vi "BLM_ManualControl.vi"() -> ()   [LabVIEW 2020]
doc: "To start rotations:\n\nSelect The Motor (BLM) address\nRun this VI\nClick Test connection button\nClick INITIALIZE button \n (It is assumed that a BLM controller should be initialized only once: immediately after it is turned on. \n E.g., usually there is no need to initialize if you rebooted computer, but kept the motor controller on,\n the motor was connected to the controller and you wish to continue using current position counting. \n Initialization occurs only if the current motor position is equal to zero.) \nClick READ BLM position button\nSelect desired MODE, SPEED, and Distance (or Final Position, depends on the MODE) value\nClick RUN BLM button\n\nSET POSITION button does not affect actual sample/motor position, but changes the position value\nin the controller memory. Thus, it allows to assign any value to the current motor position.\n\nSee also:\nhttps://opswiki.magnet.fsu.edu/wiki/pages/K7Q8u4C4s9/Rotating_probes_equipped_with_Brushless_Motors_BLMs.html\n\nNHMFL; A.Suslov; Feb 2012; updated Aug 2016"
panel:
  out "Error Out":errorcluster {"code" format="%.0x"}
  in  "MODE:":enum32{"ABSOLUTE", "INCREMENTAL"}(radio)=enum."INCREMENTAL"
  in  "Read Position":bool
  out "Test Results":string
  in  "Test Connection":bool
  out "BLM Position":dbl caption="BLM position\nincrement 0.045 \n (deg of BLM)" format="%.3f"
  in  "Parameter changed":bool
  in  "stop":bool
  in  "Set Position":bool
  in  "INITIALIZE":bool
  in  "Run":bool
  in  "New position":dbl caption="Distance:\nincrement 0.045 \n (deg of BLM)" step=0.045 format="%#.3g"
  in  "SPEED (rot/sec)\nincrement .0042":dbl=0.0294 min=0.0042 max=0.42 step=0.0042
  in  "MOTOR (BLM) Address":refnum<visa-resource-name>
  # "Select The Motor (BLM) address\nRun this VI\nClick Test connection button\nClick  INITIALIZE button \nClick  READ BLM position button\nSelect desired MODE, SPEED, and\n         Distance (or Final Position)\nClick RUN BLM button\n\nMore Help at File-> VI Propeties->\nDocumentation\nand Operations Wiki"
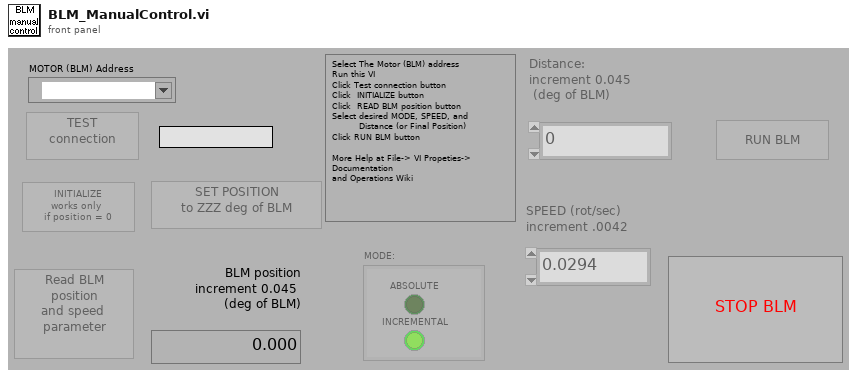
[diagram p1: front panel]
types:
  T1 = enum8{"Enabled", "Disabled", "Disabled and Grayed Out"}
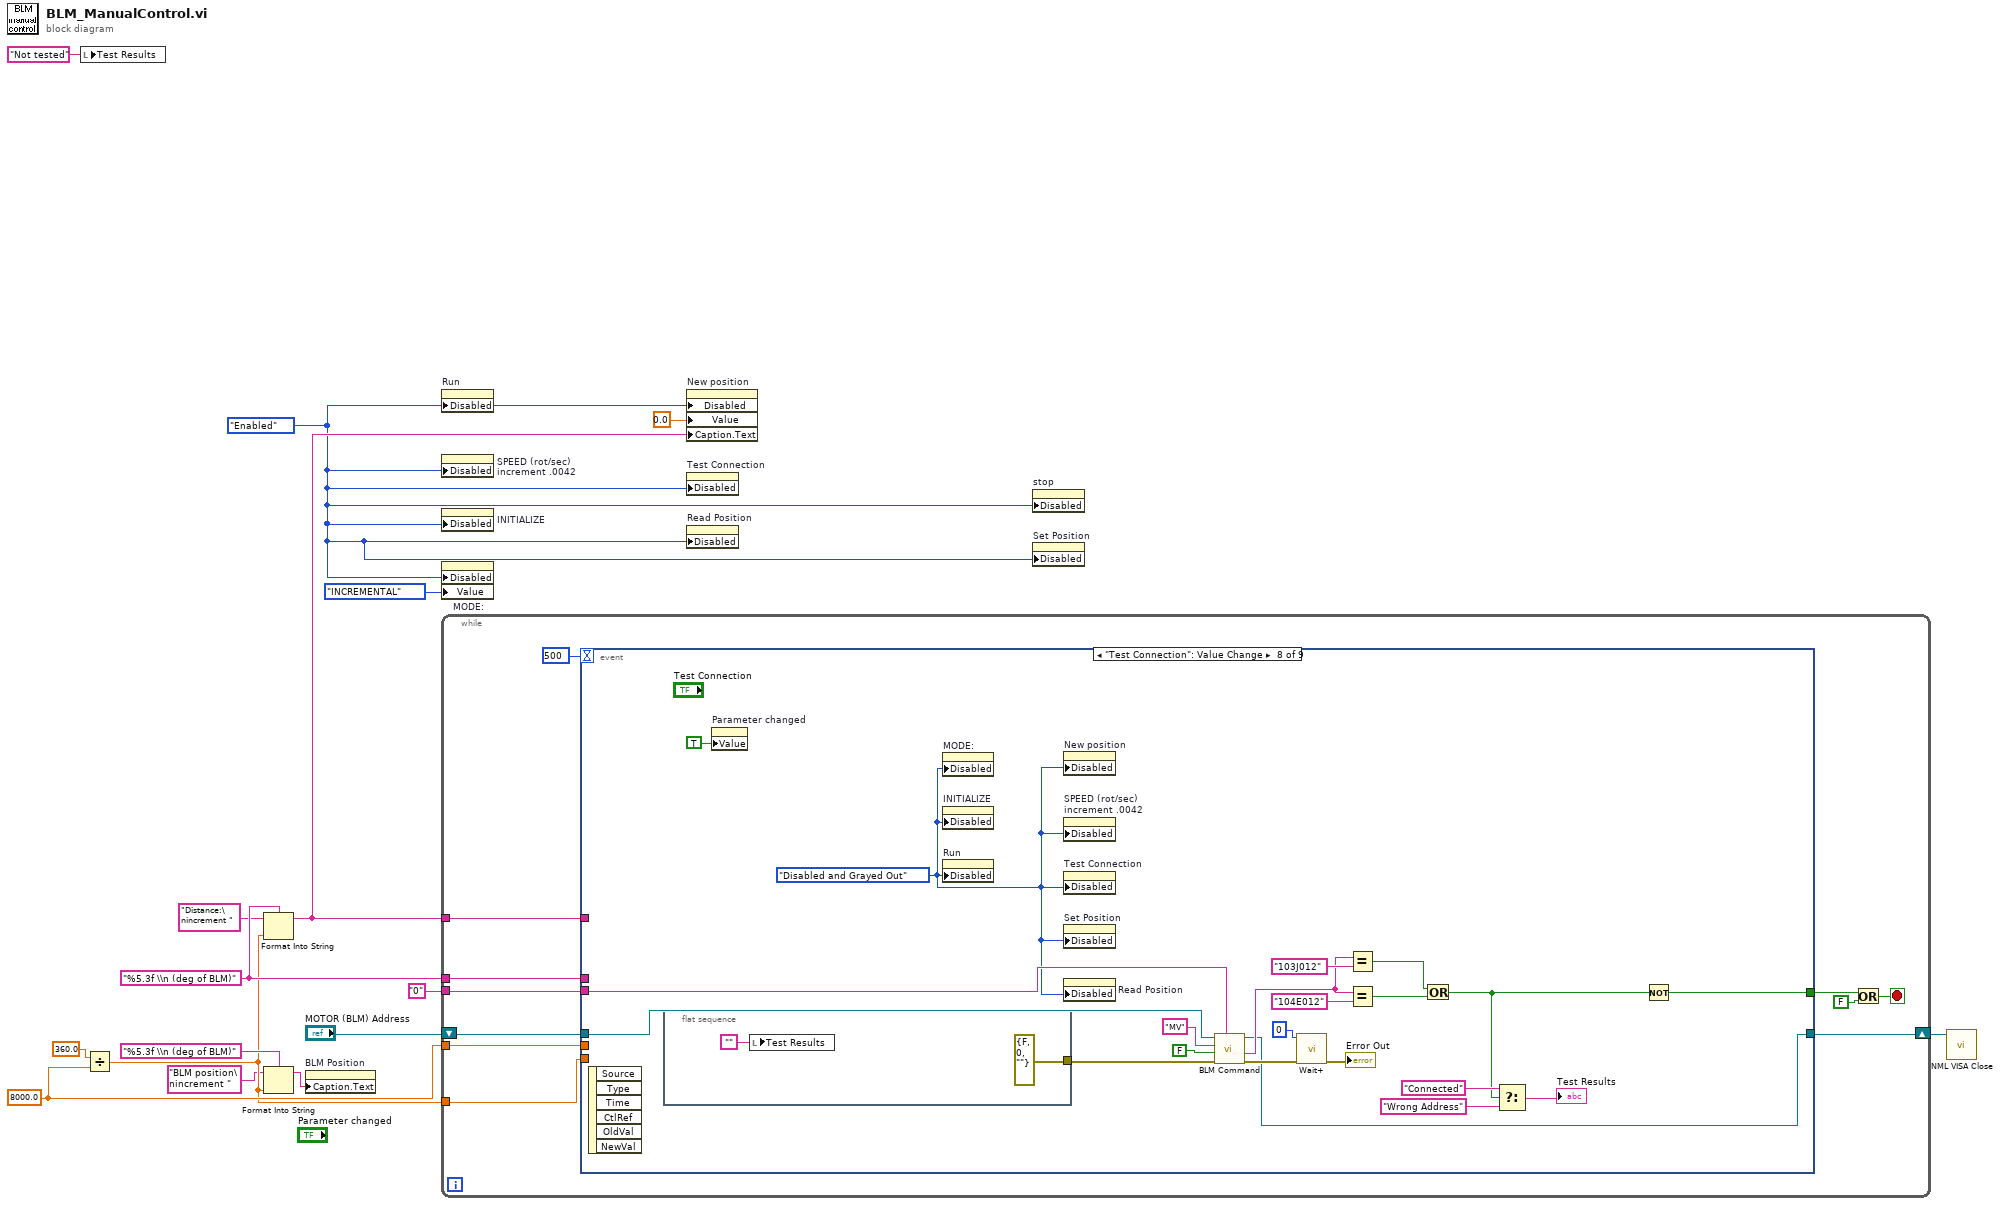
[diagram p0: block diagram]
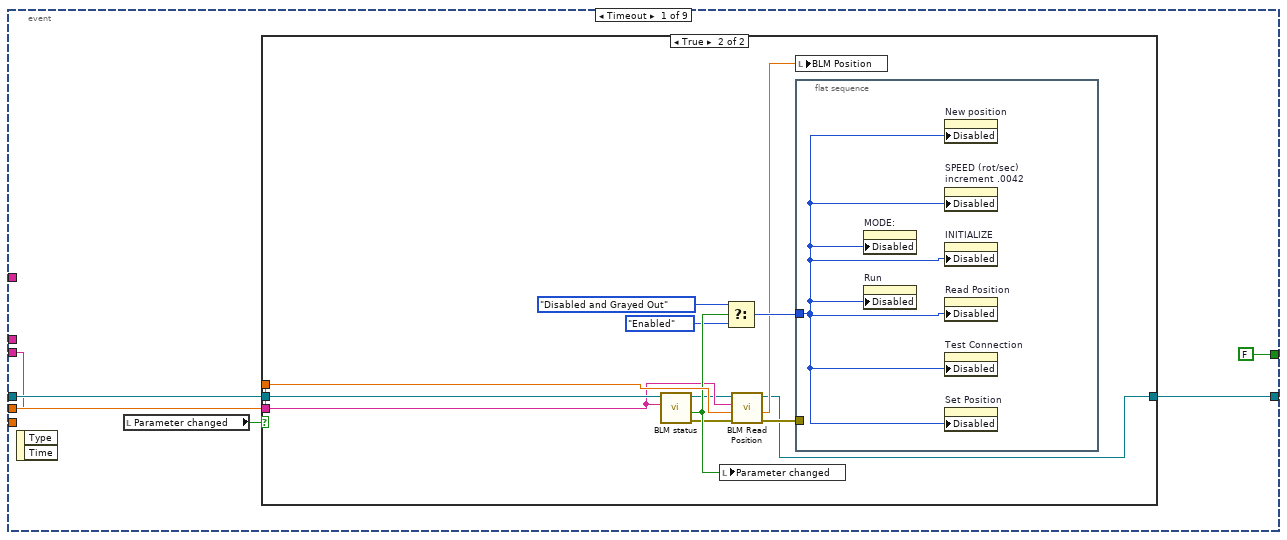
[diagram p2: hidden frame]
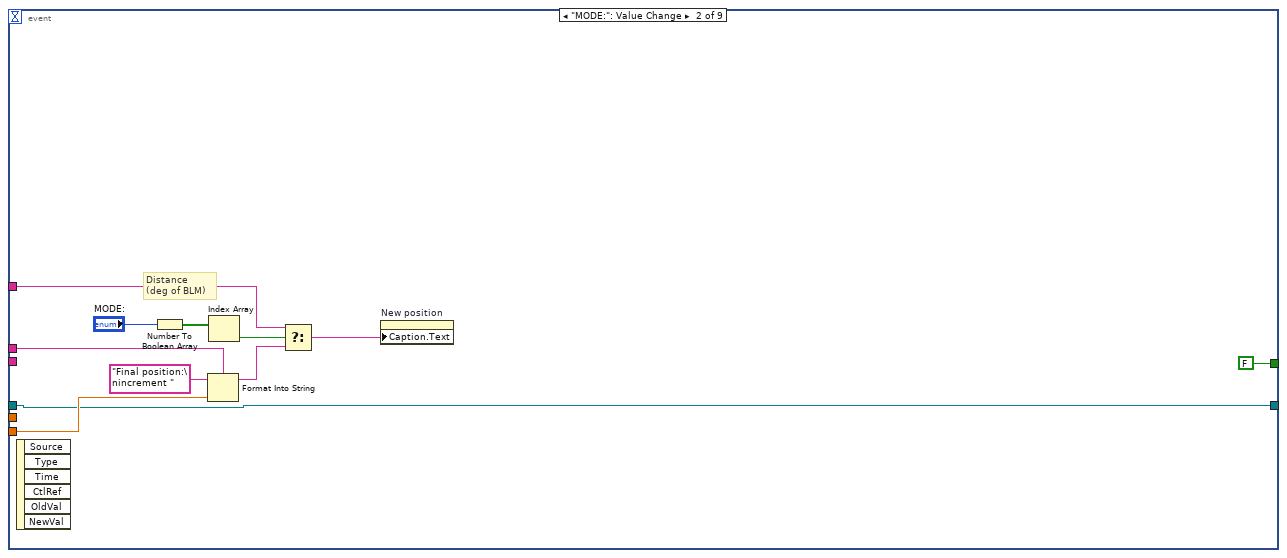
[diagram p4: hidden frame]
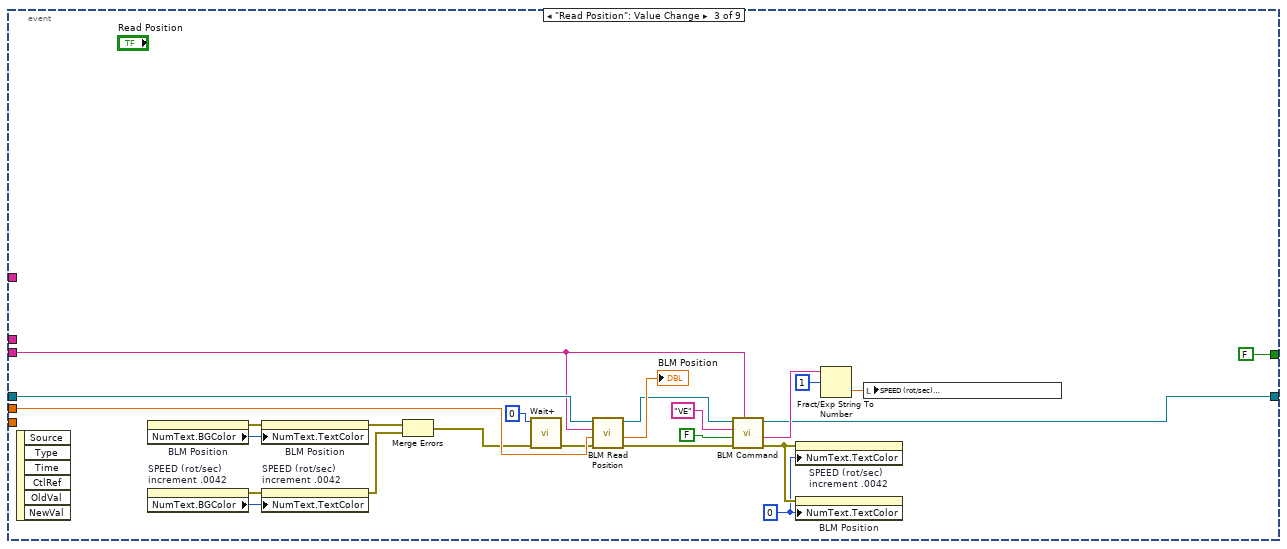
[diagram p5: hidden frame]
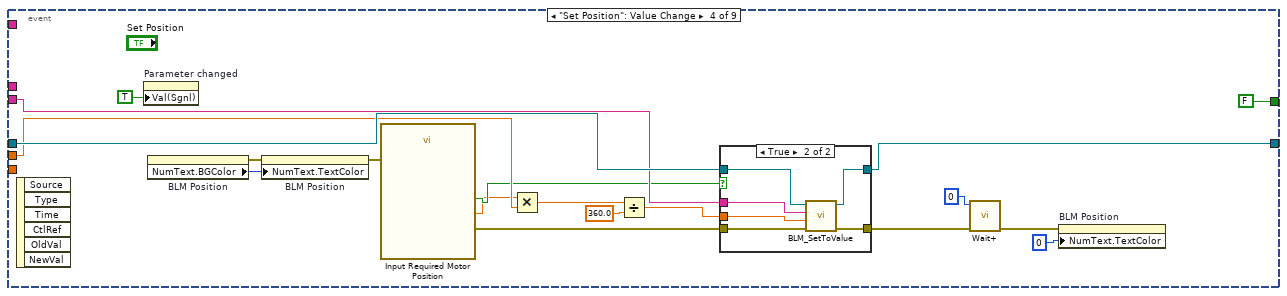
[diagram p6: hidden frame]
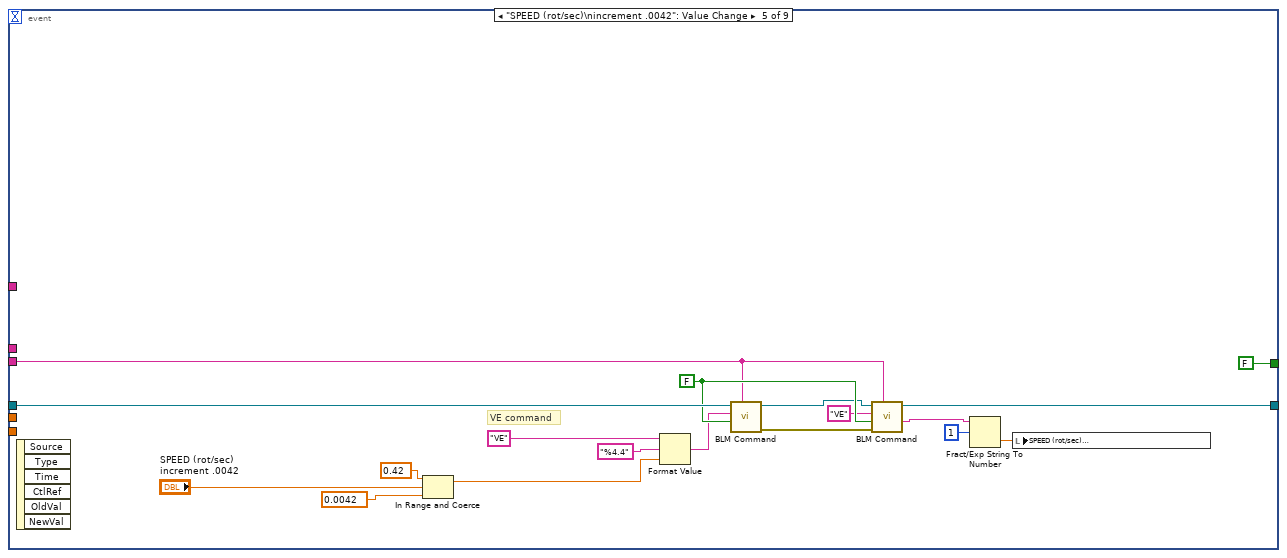
[diagram p8: hidden frame]
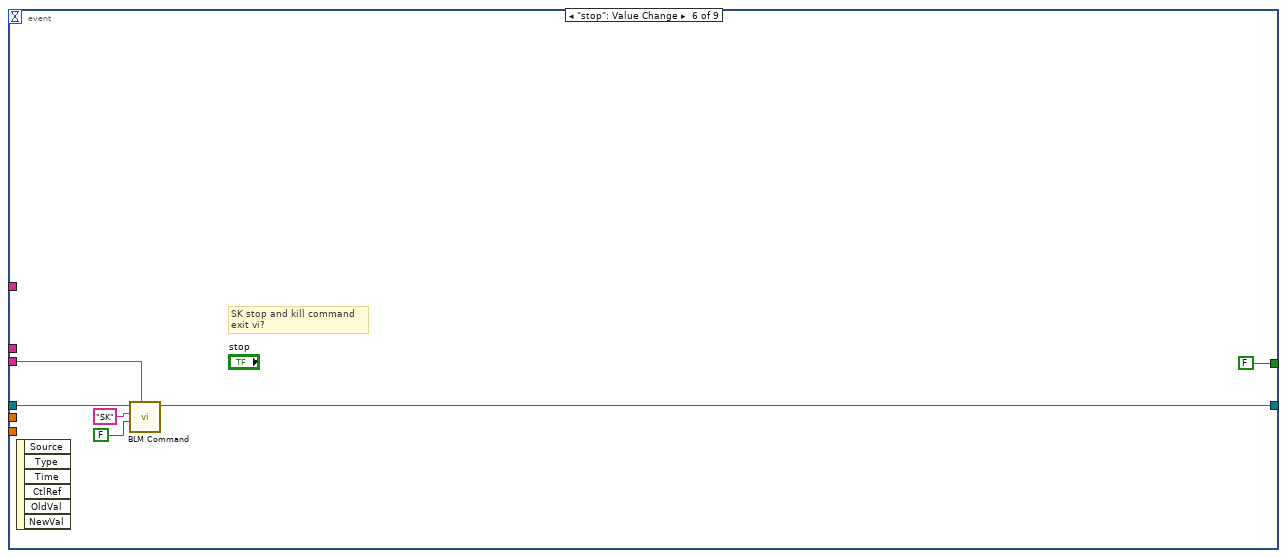
[diagram p9: hidden frame]
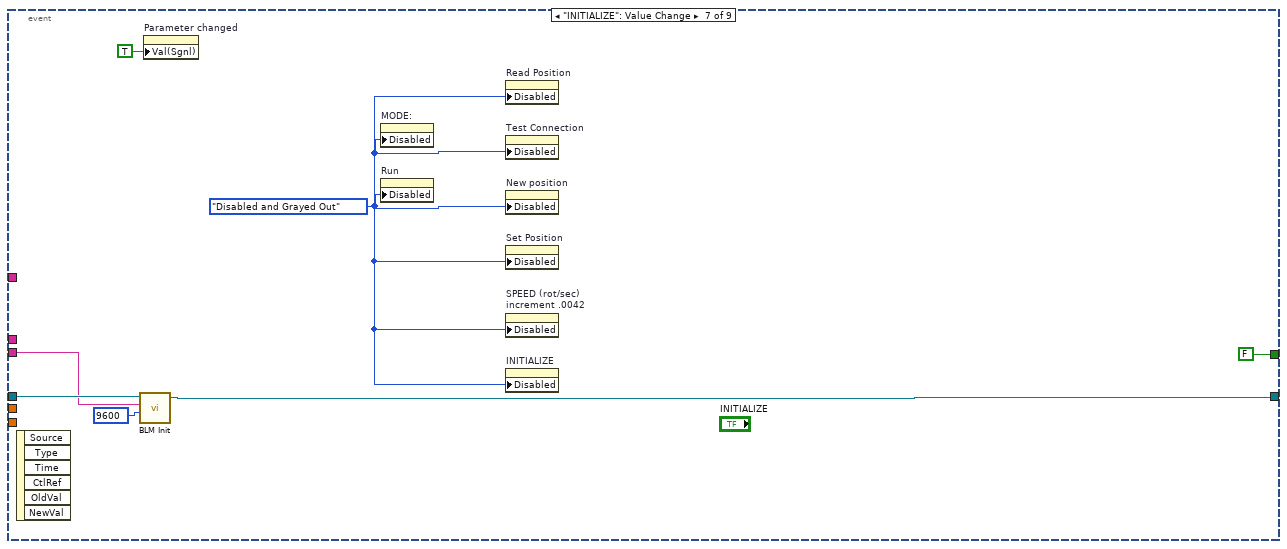
[diagram p10: hidden frame]
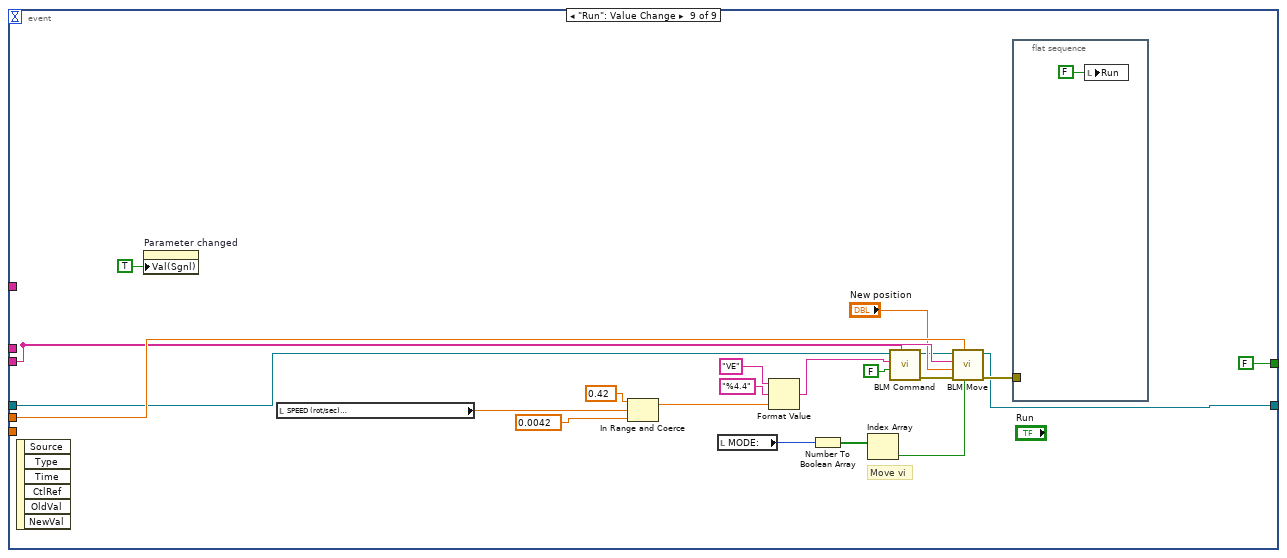
[diagram p11: hidden frame]
diagram:
  w3 = T1."Enabled" ("Disabled")
  w9 = "%5.3f \\n (deg of BLM)" ("format string")
  w11 = 8000.0 ("Steps/rot")
  n1 = local write "Test Results"("Not tested" ("s? t:f")) -> ()
  n2 = Divide(x=360.0, y=w11) -> (x/y=w6:dbl)
  n3 = Format Into String(format string=w9, initial string="Distance:\nincrement " ("Label.Text"), w6) -> (resulting string=w10:string)  [unwired: 1 in, 1 out]
  n4 = Format Into String(format string="%5.3f \\n (deg of BLM)", initial string="BLM position\nincrement ", w6) -> (resulting string=w7:string)  [unwired: 1 in, 1 out]
  n5 = property on="BLM Position" class="DigNum (strict)"("Caption.Text"=w7) -> ()  [unwired: 2 in, 2 out]
  n6 = property on="Run" class="Bool (strict)"("Disabled"=w3) -> ()  [unwired: 2 in, 2 out]
  n7 = property on="SPEED (rot/sec)\nincrement .0042" class="DigNum (strict)"("Disabled"=w3) -> ()  [unwired: 2 in, 2 out]
  n8 = property on="INITIALIZE" class="Bool"("Disabled"=w3) -> ()  [unwired: 2 in, 2 out]
  n9 = property on="MODE:" class="RadioBtnsControl (strict)"("Disabled"=w3, "Value"=enum32{"ABSOLUTE", "INCREMENTAL"}."INCREMENTAL" ("MODE:")) -> ()  [unwired: 2 in, 2 out]
  n10 = while {
    tunnel: w11 -> [w27]
    tunnel: w10 -> [w21]
    tunnel: "0" ("Motor Address") -> [w20]
    tunnel: w6 -> [w19]
    tunnel: w9 -> [w18]
    shift-right: [w17] -> w1
    shift-left: "MOTOR (BLM) Address" -> [w26]
    stop <- w23 stop-if-true
    n11 = event shown="[7] \"Test Connection\": Value Change" {
      selector: _ -> [_ _ _ _ _ _ _ _ _]
      dyn-events: _ -> [_ _ _ _ _ _ _ _ _]
      timeout: 500 -> [_ _ _ _ _ _ _ _ _]
      tunnel: w27 -> [w32 _ w82 w98 _ _ _ _ w184]
      tunnel: w26 -> [w33 w48 w81 w101 w127 w133 w139 w161 w183]
      tunnel: [FALSE FALSE FALSE FALSE FALSE FALSE FALSE w159 FALSE] -> w22
      tunnel: w21 -> [_ w57 _ _ _ _ _ _ _]
      tunnel: w20 -> [w30 _ w80 w99 w123 w130 w137 w157 w181]
      tunnel: w19 -> [_ w51 _ _ _ _ _ _ _]
      tunnel: w18 -> [_ w50 _ _ _ _ _ _ _]
      tunnel: [w28 w48 w59 w83 w110 w128 w134 w141 w164] -> w17
      event Timeout {
        n12 = event-data() -> ()  [unwired: 1 in, 2 out]
        n13 = local read "Parameter changed"() -> (w31:bool)
        n14 = case shown="True" w31 {
          tunnel: w33 -> [w34 w46]
          tunnel: w32 -> [_ w45]
          tunnel: w30 -> [_ w41]
          tunnel: [w34 w36] -> w28
          frame False {
          }
          frame True {
            n15 = call "BLM status.vi"("Motor Address"=w41, "Port Address"=w46) -> ("error out"=w40:errorcluster, "Motor is moving"=w44:bool, "Port Address Out"=w35:refnum<visa-resource-name>)  [unwired: 3 in]
            n16 = local write "Parameter changed"(w44) -> ()
            n17 = Select(t=T1."Disabled and Grayed Out" ("Disabled"), s=w44, f=T1."Enabled" ("Disabled")) -> (s? t:f=w43:T1)
            n18 = call "BLM Read Position.vi"("error in (no error)"=w40, "Steps/rot"=w45, "Motor Address"=w41, "Port Address"=w35) -> ("error out"=w39:errorcluster, "Response"=w42:dbl, "Port Address Out"=w36:refnum<visa-resource-name>)  [unwired: 1 out]
            n19 = local write "BLM Position"(w42) -> ()
            n20 = flat-sequence {
              tunnel: w43 -> [w47]
              tunnel: w39 -> [_]
              frame #0 {
                n21 = property on="MODE:" class="RadioBtnsControl (strict)"("Disabled"=w47) -> ()  [unwired: 2 in, 2 out]
                n22 = property on="Run" class="Bool (strict)"("Disabled"=w47) -> ()  [unwired: 2 in, 2 out]
                n23 = property on="New position" class="DigNum (strict)"("Disabled"=w47) -> ()  [unwired: 2 in, 2 out]
                n24 = property on="SPEED (rot/sec)\nincrement .0042" class="DigNum (strict)"("Disabled"=w47) -> ()  [unwired: 2 in, 2 out]
                n25 = property on="INITIALIZE" class="Bool"("Disabled"=w47) -> ()  [unwired: 2 in, 2 out]
                n26 = property on="Read Position" class="Bool"("Disabled"=w47) -> ()  [unwired: 2 in, 2 out]
                n27 = property on="Test Connection" class="Bool"("Disabled"=w47) -> ()  [unwired: 2 in, 2 out]
                n28 = property on="Set Position" class="Bool"("Disabled"=w47) -> ()  [unwired: 2 in, 2 out]
              }
            }
          }
        }
      }
      event "MODE:": Value Change {
        # "Distance  \n(deg of BLM)"
        n29 = event-data() -> ()  [unwired: 1 in, 6 out]
        n30 = Number To Boolean Array(number="MODE:") -> (Boolean array=w55:bool[])
        n31 = Format Into String(format string=w50, initial string="Final position:\nincrement " ("f"), w51) -> (resulting string=w53:string)  [unwired: 1 in, 1 out]
        n32 = Index Array(array=w55) -> (element=w54:bool)  [unwired: 1 in]
        n33 = Select(t=w57, s=w54, f=w53) -> (s? t:f=w58:string)
        n34 = property on="New position" class="DigNum (strict)"("Caption.Text"=w58) -> ()  [unwired: 2 in, 2 out]
      }
      event "Read Position": Value Change {
        w67 = u32 0 ("Numeric Text.Text Colors:Text Color")
        n35 = event-data() -> ()  [unwired: 1 in, 6 out]
        n36 = property on="BLM Position" class="DigNum (strict)"() -> (error out=w61:errorcluster, "NumText.BGColor"=w66:u32)  [unwired: 2 in, 1 out]
        n37 = property on="SPEED (rot/sec)\nincrement .0042" class="DigNum (strict)"() -> (error out=w62:errorcluster, "NumText.BGColor"=w65:u32)  [unwired: 2 in, 1 out]
        n38 = property on="BLM Position" class="DigNum (strict)"(error in=w61, "NumText.TextColor"=w66) -> (error out=w64:errorcluster)  [unwired: 1 in, 1 out]
        n39 = property on="SPEED (rot/sec)\nincrement .0042" class="DigNum (strict)"(error in=w62, "NumText.TextColor"=w65) -> (error out=w63:errorcluster)  [unwired: 1 in, 1 out]
        n40 = Merge Errors(w64, w63) -> (w68:errorcluster)
        n41 = call "Wait+.vi"("Error In"=w68, "milliseconds to wait"=u32 0 ("millisecond timer value")) -> ("Error Out"=w70:errorcluster)  [unwired: 4 in, 1 out]
        n42 = call "BLM Read Position.vi"("error in (no error)"=w70, "Steps/rot"=w82, "Motor Address"=w80, "Port Address"=w81) -> ("error out"=w72:errorcluster, "Response"=→"BLM Position":dbl, "Port Address Out"=w60:refnum<visa-resource-name>)  [unwired: 1 out]
        n43 = call "BLM Command.vi"("Motor Address"=w80, "error in (no error)"=w72, "Read Echo?"=FALSE, "Command"="VE", "Port Address"=w60) -> ("error out"=w78:errorcluster, "Response"=w75:string, "Port Address Out"=w59:refnum<visa-resource-name>)  [unwired: 1 in, 2 out]
        n44 = property on="SPEED (rot/sec)\nincrement .0042" class="DigNum (strict)"(error in=w78, "NumText.TextColor"=w67) -> ()  [unwired: 1 in, 2 out]
        n45 = property on="BLM Position" class="DigNum (strict)"(error in=w78, "NumText.TextColor"=w67) -> ()  [unwired: 1 in, 2 out]
        n46 = Fract/Exp String To Number(string=w75, offset=1) -> (number=w73:dbl)  [unwired: 2 in, 1 out]
        n47 = local write "SPEED (rot/sec)\nincrement .0042"(w73) -> ()
      }
      event "Set Position": Value Change {
        n48 = event-data() -> ()  [unwired: 1 in, 6 out]
        n49 = property on="Parameter changed" class="Bool (strict)"("Val(Sgnl)"=TRUE ("Value (Signaling)")) -> ()  [unwired: 2 in, 2 out]
        n50 = property on="BLM Position" class="DigNum (strict)"() -> (error out=w84:errorcluster, "NumText.BGColor"=w93:u32)  [unwired: 2 in, 1 out]
        n51 = property on="BLM Position" class="DigNum (strict)"(error in=w84, "NumText.TextColor"=w93) -> (error out=w94:errorcluster)  [unwired: 1 in, 1 out]
        n52 = call "Input Required Motor Position"("error in (no error)"=w94) -> ("Position:"=w91:dbl, "OK"=w92:bool, "error out"=w87:errorcluster)  [unwired: 16 in]
        n53 = Multiply(x=w91, y=w98) -> (x*y=w89:dbl)
        n54 = Divide(x=w89, y=360.0) -> (x/y=w90:dbl)
        n55 = case shown="True" w92 {
          tunnel: w101 -> [w102 w109]
          tunnel: w99 -> [_ w108]
          tunnel: w90 -> [_ w107]
          tunnel: [w103 w106] -> w96
          tunnel: w87 -> [w103 w105]
          tunnel: [w102 w104] -> w83
          frame False {
          }
          frame True {
            n56 = call "BLM_SetToValue.vi"("error in (no error)"=w105, "Position"=w107, "Motor Address"=w108, "Port Address"=w109) -> ("error out"=w106:errorcluster, "Port Address Out"=w104:refnum<visa-resource-name>)  [unwired: 2 in]
          }
        }
        n57 = call "Wait+.vi"("Error In"=w96, "milliseconds to wait"=u32 0) -> ("Error Out"=w95:errorcluster)  [unwired: 4 in, 1 out]
        n58 = property on="BLM Position" class="DigNum (strict)"(error in=w95, "NumText.TextColor"=u32 0 ("Numeric Text.Text Colors:Text Color")) -> ()  [unwired: 1 in, 2 out]
      }
      event "SPEED (rot/sec)\nincrement .0042": Value Change {
        w126 = FALSE
        # "VE command"
        n59 = event-data() -> ()  [unwired: 1 in, 6 out]
        n60 = In Range and Coerce(upper limit=0.42 ("x"), x="SPEED (rot/sec)\nincrement .0042", lower limit=0.0042) -> (coerced(x)=w119:dbl)  [unwired: 1 out]
        n61 = Format Value(string ("")="VE", format string="%4.4", value (0)=w119) -> (output string=w116:string)
        n62 = call "BLM Command.vi"("Motor Address"=w123, "Read Echo?"=w126, "Command"=w116, "Port Address"=w127) -> ("error out"=w124:errorcluster, "Port Address Out"=w111:refnum<visa-resource-name>)  [unwired: 2 in, 3 out]
        n63 = call "BLM Command.vi"("Motor Address"=w123, "error in (no error)"=w124, "Read Echo?"=w126, "Command"="VE", "Port Address"=w111) -> ("Response"=w113:string, "Port Address Out"=w110:refnum<visa-resource-name>)  [unwired: 1 in, 3 out]
        n64 = Fract/Exp String To Number(string=w113, offset=1) -> (number=w125:dbl)  [unwired: 2 in, 1 out]
        n65 = local write "SPEED (rot/sec)\nincrement .0042"(w125) -> ()
      }
      event "stop": Value Change {
        # "SK stop and kill command\nexit vi?"
        n66 = event-data() -> ()  [unwired: 1 in, 6 out]
        n67 = call "BLM Command.vi"("Motor Address"=w130, "Read Echo?"=FALSE, "Command"="SK", "Port Address"=w133) -> ("Port Address Out"=w128:refnum<visa-resource-name>)  [unwired: 2 in, 4 out]
      }
      event "INITIALIZE": Value Change {
        w135 = T1."Disabled and Grayed Out" ("Disabled")
        n68 = event-data() -> ()  [unwired: 1 in, 6 out]
        n69 = call "BLM Init.vi"("Baud Rate"=u32 9600, "Motor Address"=w137, "Port Address"=w139) -> ("Port Address Out"=w134:refnum<visa-resource-name>)  [unwired: 1 in, 2 out]
        n70 = property on="Parameter changed" class="Bool (strict)"("Val(Sgnl)"=TRUE ("Value (Signaling)")) -> ()  [unwired: 2 in, 2 out]
        n71 = property on="MODE:" class="RadioBtnsControl (strict)"("Disabled"=w135) -> ()  [unwired: 2 in, 2 out]
        n72 = property on="Run" class="Bool (strict)"("Disabled"=w135) -> ()  [unwired: 2 in, 2 out]
        n73 = property on="Read Position" class="Bool"("Disabled"=w135) -> ()  [unwired: 2 in, 2 out]
        n74 = property on="Test Connection" class="Bool"("Disabled"=w135) -> ()  [unwired: 2 in, 2 out]
        n75 = property on="New position" class="DigNum (strict)"("Disabled"=w135) -> ()  [unwired: 2 in, 2 out]
        n76 = property on="Set Position" class="Bool"("Disabled"=w135) -> ()  [unwired: 2 in, 2 out]
        n77 = property on="SPEED (rot/sec)\nincrement .0042" class="DigNum (strict)"("Disabled"=w135) -> ()  [unwired: 2 in, 2 out]
        n78 = property on="INITIALIZE" class="Bool"("Disabled"=w135) -> ()  [unwired: 2 in, 2 out]
      }
      event "Test Connection": Value Change {
        w156 = T1."Disabled and Grayed Out" ("Disabled")
        n79 = event-data() -> ()  [unwired: 1 in, 6 out]
        n80 = flat-sequence {
          tunnel: [errorcluster {"status"=FALSE, "code"=0, "source"=""} ("error in (no error)")] -> w147
          frame #0 {
            n81 = local write "Test Results"("" ("Response")) -> ()
          }
        }
        n82 = property on="Parameter changed" class="Bool (strict)"("Value"=TRUE ("Parameter changed")) -> ()  [unwired: 2 in, 2 out]
        n83 = property on="MODE:" class="RadioBtnsControl (strict)"("Disabled"=w156) -> ()  [unwired: 2 in, 2 out]
        n84 = property on="INITIALIZE" class="Bool"("Disabled"=w156) -> ()  [unwired: 2 in, 2 out]
        n85 = property on="Run" class="Bool (strict)"("Disabled"=w156) -> ()  [unwired: 2 in, 2 out]
        n86 = property on="New position" class="DigNum (strict)"("Disabled"=w156) -> ()  [unwired: 2 in, 2 out]
        n87 = property on="SPEED (rot/sec)\nincrement .0042" class="DigNum (strict)"("Disabled"=w156) -> ()  [unwired: 2 in, 2 out]
        n88 = property on="Test Connection" class="Bool"("Disabled"=w156) -> ()  [unwired: 2 in, 2 out]
        n89 = property on="Set Position" class="Bool"("Disabled"=w156) -> ()  [unwired: 2 in, 2 out]
        n90 = property on="Read Position" class="Bool"("Disabled"=w156) -> ()  [unwired: 2 in, 2 out]
        n91 = call "BLM Command.vi"("Motor Address"=w157, "error in (no error)"=w147, "Read Echo?"=FALSE, "Command"="MV", "Port Address"=w161) -> ("error out"=w155:errorcluster, "Response"=w144:string, "Port Address Out"=w141:refnum<visa-resource-name>)  [unwired: 1 in, 2 out]
        n92 = call "Wait+.vi"("Error In"=w155, "milliseconds to wait"=u32 0) -> ("Error Out"=→"Error Out":errorcluster)  [unwired: 4 in, 1 out]
        n93 = Equal?(x=w144, y="103J012" ("Response")) -> (x = y?=w160:bool)
        n94 = Equal?(x=w144, y="104E012" ("Response")) -> (x = y?=w143:bool)
        n95 = Or(x=w160, y=w143) -> (x .or. y?=w145:bool)
        n96 = Select(t="Connected" ("Response"), s=w145, f="Wrong Address" ("Response")) -> (s? t:f=→"Test Results":string)
        n97 = Not(x=w145) -> (.not. x?=w159:bool)
      }
      event "Run": Value Change {
        # "Move vi"
        n98 = event-data() -> ()  [unwired: 1 in, 6 out]
        n99 = property on="Parameter changed" class="Bool (strict)"("Val(Sgnl)"=TRUE ("Value (Signaling)")) -> ()  [unwired: 2 in, 2 out]
        n100 = local read "SPEED (rot/sec)\nincrement .0042"() -> (w182:dbl)
        n101 = In Range and Coerce(upper limit=0.42 ("x"), x=w182, lower limit=0.0042) -> (coerced(x)=w176:dbl)  [unwired: 1 out]
        n102 = local read "MODE:"() -> (w168:enum32{"ABSOLUTE", "INCREMENTAL"})
        n103 = Format Value(string ("")="VE", format string="%4.4", value (0)=w176) -> (output string=w172:string)
        n104 = Number To Boolean Array(number=w168) -> (Boolean array=w169:bool[])
        n105 = Index Array(array=w169) -> (element=w167:bool)  [unwired: 1 in]
        n106 = call "BLM Command.vi"("Motor Address"=w181, "Read Echo?"=FALSE, "Command"=w172, "Port Address"=w183) -> ("error out"=w180:errorcluster, "Port Address Out"=w165:refnum<visa-resource-name>)  [unwired: 2 in, 3 out]
        n107 = call "BLM Move.vi"("Mode IS:"=w167, "Steps/rot"=w184, "error in (no error)"=w180, "Position / Distance"="New position", "Motor Address"=w181, "Port Address"=w165) -> ("error out"=w179:errorcluster, "Port Address Out"=w164:refnum<visa-resource-name>)  [unwired: 2 in]
        n108 = flat-sequence {
          tunnel: w179 -> [_]
          frame #0 {
            n109 = local write "Run"(FALSE ("Run")) -> ()
          }
        }
      }
    }
    n110 = Or(x=w22, y=FALSE) -> (x .or. y?=w23:bool)
  }
  n111 = property on="New position" class="DigNum (strict)"("Disabled"=w3, "Value"=0.0 ("New position / \n distance (deg of BLM)"), "Caption.Text"=w10) -> ()  [unwired: 2 in, 2 out]
  n112 = property on="Test Connection" class="Bool"("Disabled"=w3) -> ()  [unwired: 2 in, 2 out]
  n113 = property on="Read Position" class="Bool"("Disabled"=w3) -> ()  [unwired: 2 in, 2 out]
  n114 = property on="stop" class="Bool"("Disabled"=w3) -> ()  [unwired: 2 in, 2 out]
  n115 = property on="Set Position" class="Bool"("Disabled"=w3) -> ()  [unwired: 2 in, 2 out]
  n116 = call "NML VISA Close.vi"("VISA resource name"=w1) -> ()  [unwired: 10 in, 1 out]
